vi "Cast Boolean to Variant.vi"(8 "error in (no error)":errorcluster, 11 "JSON Boolean in":refnum<class "JSON Boolean.lvclass">) -> (0 "error out":errorcluster, 2 "Variant":variant)   [LabVIEW 2015]
doc: "Converts the given JSON Boolean to a variant"
uses:
  Read value (Boolean).vi
  JSON Boolean.lvclass
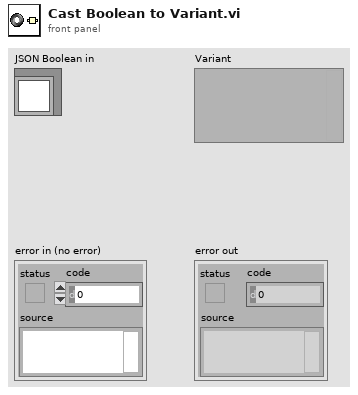
[diagram p1: front panel]
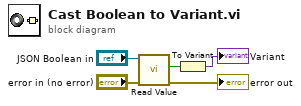
[diagram p0: block diagram]
diagram:
  n1 = call-poly "Read Value.vi"("error in (no error)"="error in (no error)", "JSON String in"="JSON Boolean in") -> ("error out"=→"error out":errorcluster, "value"=w1:bool)  [unwired: 7 in, 1 out]
  n2 = To Variant(anything=w1) -> (Variant=→"Variant":variant)
